vi "Finish.vi"   [LabVIEW 2020]
doc: "This VI is called just before exiting. It is expected to close I/O refnum, save collected data, etc."
uses:
  <vilib>/Rock Robotics/WPI/Utilities/WPI_GetSetVariantRefNum.vi
types:
  T1 = typedef "WPI_JoystickDevRef.ctl" = cluster{"Device":T2}
  T2 = typedef "WPI_JoystickDeviceEnum.ctl" = enum16{"USB 0", "USB 1", "USB 2", "USB 3", "USB 4", "USB 5"}
  T3 = typedef "WPI_MotorControlDeviceRef.ctl" = cluster{"DeviceStatus":errorcluster, "Type":T4, "PWM":cluster{"PWM Channel":T5, "DeadBand":T6}, "CAN":cluster{"Device Number":u8, "SetOutput VI Ref":variant, "GetOutput VI Ref":variant, "Enable VI Ref":variant, "Disable VI Ref":variant, "Data":variant}, "Invert":bool, "DIO PWM":cluster{"PWM \"Enable\" Channel":T5, "DIOChannel":T7, "PWM Rate":dbl}}
  T4 = typedef "WPI_MotorControlType.ctl" = enum16{"PWM", "CAN", "DIO PWM"}
  T5 = typedef "FPGA_DIOPWMChannel.ctl" = enum8{"PWM 0", "PWM 1", "PWM 2", "PWM 3", "PWM 4", "PWM 5", "PWM 6", "PWM 7", "PWM 8", "PWM 9", "PWM MXP 0", "PWM MXP 1", "PWM MXP 2", "PWM MXP 3", "PWM MXP 4", "PWM MXP 5", "PWM MXP 6", "PWM MXP 7", "PWM MXP 8", "PWM MXP 9", "Invalid"}
  T6 = typedef "WPI_PWMDeadband.ctl" = cluster{"Name":string, "maxPositivePwm":i32, "minPositivePwm":i32, "centerPwm":i32, "maxNegativePwm":i32, "minNegativePwm":i32, "angularRange":u16}
  T7 = typedef "FPGA_DIOChannel.ctl" = enum8{"DIO 0", "DIO 1", "DIO 2", "DIO 3", "DIO 4", "DIO 5", "DIO 6", "DIO 7", "DIO 8", "DIO 9", "DIO MXP 0", "DIO MXP 1", "DIO MXP 2", "DIO MXP 3", "DIO MXP 4", "DIO MXP 5", "DIO MXP 6", "DIO MXP 7", "DIO MXP 8", "DIO MXP 9", "DIO MXP 10", "DIO MXP 11", "DIO MXP 12", "DIO MXP 13", "DIO MXP 14", "DIO MXP 15", "SPI Port CS1", "SPI Port CS2", "SPI Port CS3", "SPI Port MISO", "SPI Port MOSI", "Invalid"}
  T8 = typedef "WPI_GyroDevRef.ctl" = cluster{"DevStatus":errorcluster, "Analog Channel":T9, "Gain (VoltsPerDegree/Second)":dbl, "Gyro Type":enum16{"Analog", "XRS450"}, "Handle":i32, "SPI Bus":T10, "Device Found":bool, "Sample Rate":dbl, "Calibrate On Open":bool, "Offset":dbl}
  T9 = typedef "FPGA_AIChannel.ctl" = enum8{"AI 0", "AI 1", "AI 2", "AI 3", "AI MXP 0", "AI MXP 1", "AI MXP 2", "AI MXP 3", "Invalid"}
  T10 = typedef "spi_bus.ctl" = enum16{"SPI On-Board, CS0", "SPI On-Board, CS1", "SPI On-Board, CS2", "SPI On-Board, CS3", "SPI MXP", "Invalid"}
  T11 = typedef "WPI_EncoderDevRef.ctl" = cluster{"DevStatus":errorcluster, "EncoderIndex":T12, "CounterIndex":T13, "DistancePerCount":dbl, "Decoding Type":T14}
  T12 = typedef "FPGA_EncoderIdx.ctl" = enum8{"Enc 0", "Enc 1", "Enc 2", "Enc 3", "Enc 4", "Enc 5", "Enc 6", "Enc 7", "Invalid"}
  T13 = typedef "FPGA_CounterCtrSystemIndex.ctl" = enum8{"Ctr 0", "Ctr 1", "Ctr 2", "Ctr 3", "Ctr 4", "Ctr 5", "Ctr 6", "Ctr 7", "Invalid"}
  T14 = typedef "WPI_EncoderType.ctl" = enum16{"1x", "2x", "4x"}
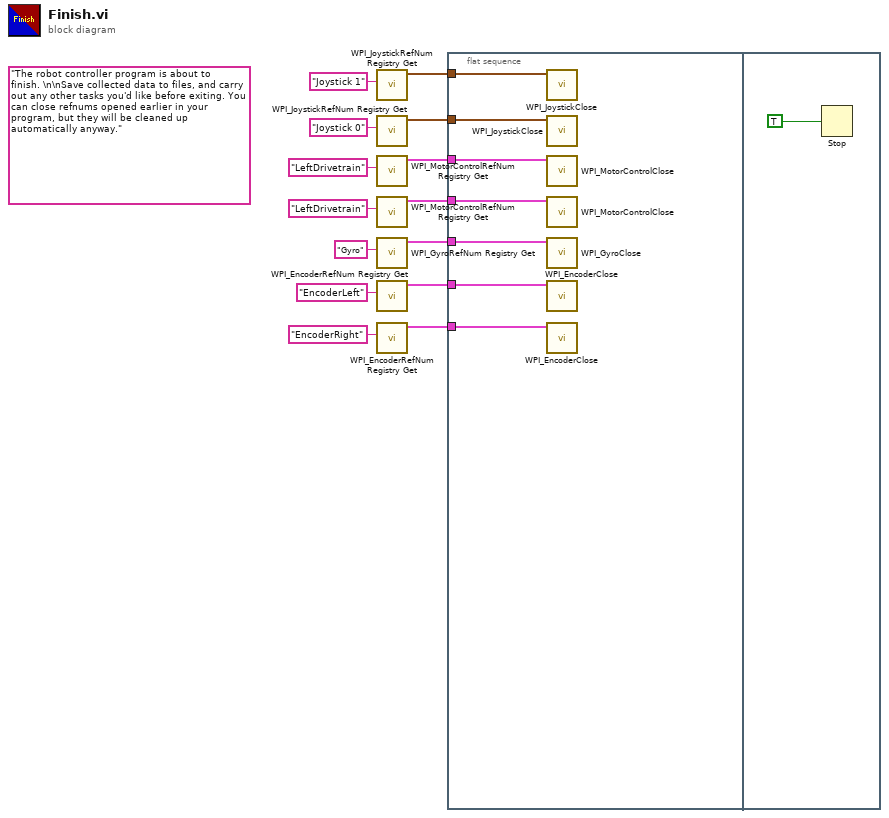
[diagram p0: block diagram]
diagram:
  (unwired) "The robot controller program is about to finish. \n\nSave collected data to files, and carry out any other tasks you'd like before exiting. You can close refnums opened earlier in your program, but they will be cleaned up automatically anyway."
  n1 = call <vilib>:"WPI_JoystickRefNum Registry Get.vi"("refnum name"="Joystick 1") -> ("JoystickDevRef"=w7:T1)  [unwired: 1 in, 9 out]
  n2 = call <vilib>:"WPI_JoystickRefNum Registry Get.vi"("refnum name"="Joystick 0") -> ("JoystickDevRef"=w13:T1)  [unwired: 1 in, 9 out]
  n3 = call <vilib>:"WPI_MotorControlRefNum Registry Get.vi"("refnum name"="LeftDrivetrain") -> ("MotorControlDevRef"=w11:T3)  [unwired: 9 in, 1 out]
  n4 = call <vilib>:"WPI_MotorControlRefNum Registry Get.vi"("refnum name"="LeftDrivetrain") -> ("MotorControlDevRef"=w9:T3)  [unwired: 9 in, 1 out]
  n5 = call <vilib>:"WPI_GyroRefNum Registry Get.vi"("refnum name"="Gyro") -> ("GyroDevRef"=w5:T8)  [unwired: 9 in, 1 out]
  n6 = call <vilib>:"WPI_EncoderRefNum Registry Get.vi"("refnum name"="EncoderLeft") -> ("EncoderDevRef"=w6:T11)  [unwired: 9 in, 1 out]
  n7 = call <vilib>:"WPI_EncoderRefNum Registry Get.vi"("refnum name"="EncoderRight") -> ("EncoderDevRef"=w3:T11)  [unwired: 9 in, 1 out]
  n8 = flat-sequence {
    tunnel: w13 -> [w21]
    tunnel: w11 -> [w20]
    tunnel: w9 -> [w19]
    tunnel: w7 -> [w18]
    tunnel: w6 -> [w17]
    tunnel: w5 -> [w16]
    tunnel: w3 -> [w15]
    frame #0 {
      n9 = call <vilib>:"WPI_JoystickClose.vi"("JoystickDevRef"=w18) -> ()  [unwired: 11 out]
      n10 = call <vilib>:"WPI_JoystickClose.vi"("JoystickDevRef"=w21) -> ()  [unwired: 11 out]
      n11 = call <vilib>:"WPI_MotorControlClose.vi"("MotorControlDevRef"=w20) -> ()  [unwired: 10 in, 1 out]
      n12 = call <vilib>:"WPI_MotorControlClose.vi"("MotorControlDevRef"=w19) -> ()  [unwired: 10 in, 1 out]
      n13 = call <vilib>:"WPI_GyroClose.vi"("GyroDevRef"=w16) -> ()  [unwired: 10 in, 1 out]
      n14 = call <vilib>:"WPI_EncoderClose.vi"("EncoderDevRef"=w17) -> ()  [unwired: 10 in, 1 out]
      n15 = call <vilib>:"WPI_EncoderClose.vi"("EncoderDevRef"=w15) -> ()  [unwired: 10 in, 1 out]
    }
    frame #1 {
      n16 = Stop(stop? (T)=TRUE ("Quit")) -> ()
    }
  }
